vi "Destroy.vi"(0 "reference in":refnum<class "G#Template.lvclass">, 5 "error in (no error)":errorcluster) -> (14 "reference out":refnum<class "G#Template.lvclass">, 19 "error out":errorcluster)   [LabVIEW 2017, in "G#Template.lvclass"]
doc: "Destructor."
uses:
  <vilib>/addons/_AddQ/G#Templates/G#Template/G#Template.lvclass
  <vilib>/addons/_AddQ/G#Object/G#Object.lvclass
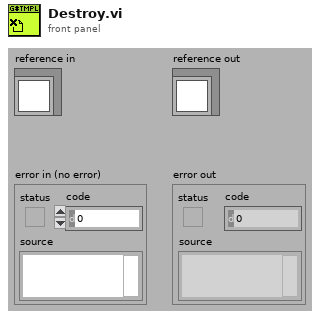
[diagram p1: front panel]
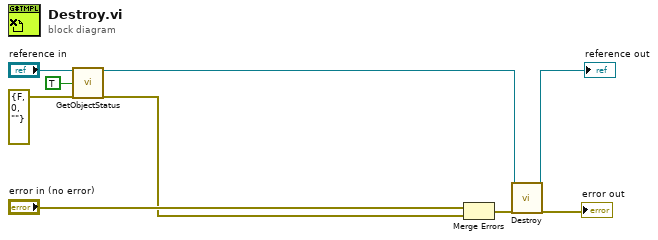
[diagram p0: block diagram]
diagram:
  n1 = call-dynamic "GetObjectStatus.vi"("reference in"="reference in", "simple info (F)"=TRUE ("simple info"), "error in (no error)"=errorcluster {"status"=FALSE, "code"=0, "source"=""}) -> ("reference out"=w1:refnum<class "G#Template.lvclass">, "error out"=w2:errorcluster)  [unwired: 5 in, 10 out]
  n2 = Merge Errors("error in (no error)", w2) -> (w8:errorcluster)
  n3 = call-parent "Destroy.vi"("reference in"=w1, "error in (no error)"=w8) -> ("reference out"=→"reference out":refnum<class "G#Template.lvclass">, "error out"=→"error out":errorcluster)  [unwired: 16 in]
